vi "Teleop.vi"(10 "Match Info":T1={"Autonomous Elapsed Seconds"=0.0, "TeleOp Elapsed Seconds"=0.0, "Disabled Elapsed Seconds"=0.0, "Visited Autonomous"=FALSE, "Visited TeleOp"=FALSE, "Visited Disabled"=FALSE, "Autonomous Settings"={"Autonomous Style"=enum."Independent", "VI Refnum"=refnum}}, 11 "Call Context":T2) -> ()   [LabVIEW 2012]
doc: "This VI is called for each TeleOp packet received from the DS where the robot is not disabled. It is often used to read from the joysticks and update I/O or to update setpoints for timed control loops. It should complete and return within 20 milliseconds or it may miss DS packets."
uses:
  <vilib>/Rock Robotics/WPI/DriverStation/WPI_DriverStationDerivedRobotMode.ctl
  <vilib>/Rock Robotics/WPI/DriverStation/WPI_DriverStationMatch Info.ctl
  <vilib>/Rock Robotics/WPI/Relay/WPI_RelayValue.ctl
  Robot Global Data.vi
  <vilib>/Rock Robotics/WPI/Joystick/WPI_JoystickGetSetRefNum.vi
panel:
  in  "Numeric":dbl=0.87
  in  "Ext Const":dbl=0.5
  in  "Dep Const":dbl=1.0
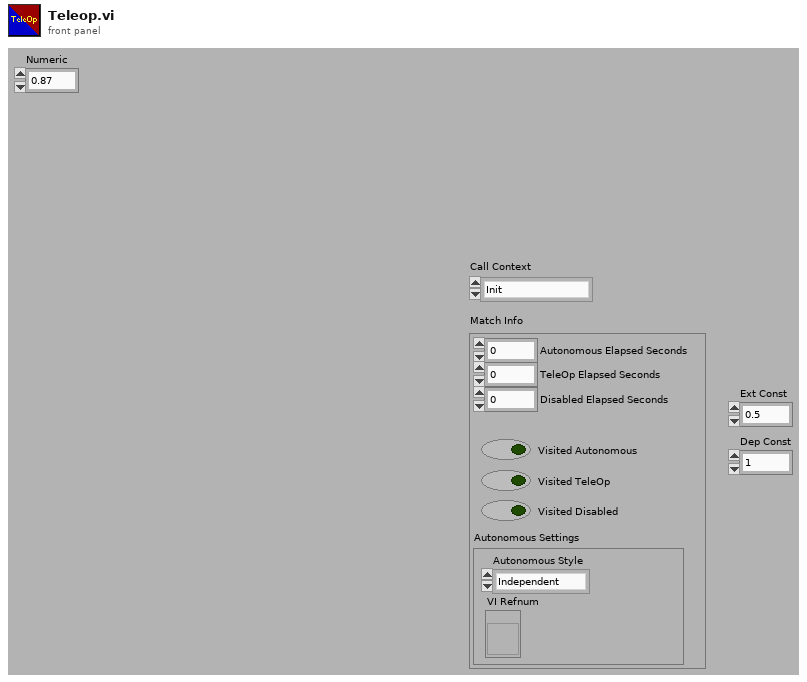
[diagram p1: front panel]
types:
  T1 = typedef "WPI_DriverStationMatch Info.ctl" = cluster{"Autonomous Elapsed Seconds":dbl, "TeleOp Elapsed Seconds":dbl, "Disabled Elapsed Seconds":dbl, "Visited Autonomous":bool, "Visited TeleOp":bool, "Visited Disabled":bool, "Autonomous Settings":cluster{"Autonomous Style":enum16{"Iterative", "Independent"}, "VI Refnum":refnum<vi>}}
  T2 = typedef "WPI_DriverStationDerivedRobotMode.ctl" = enum16{"Init", "Execute", "Stop"}
  T3 = typedef "WPI_RelayValue.ctl" = enum16{"Off", "On", "Forward", "Reverse"}
  T4 = cluster{"Driver Station Digital Input (1-8)[0]":bool, "Driver Station Digital Input (1-8)[1]":bool, "Driver Station Digital Input (1-8)[2]":bool, "Driver Station Digital Input (1-8)[3]":bool, "Driver Station Digital Input (1-8)[4]":bool, "Driver Station Digital Input (1-8)[5]":bool, "Driver Station Digital Input (1-8)[6]":bool, "Driver Station Digital Input (1-8)[7]":bool, "Driver Station Digital Input (1-8)[8]":bool}
  T5 = typedef "WPI_DigitalInputDevRef.ctl" = cluster{"DevStatus":errorcluster, "DIO Channel":T6, "Digital Module":T7}
  T6 = typedef "FPGA_DIOChannel.ctl" = enum8{"DIO 1", "DIO 2", "DIO 3", "DIO 4", "DIO 5", "DIO 6", "DIO 7", "DIO 8", "DIO 9", "DIO 10", "DIO 11", "DIO 12", "DIO 13", "DIO 14", "Invalid"}
  T7 = typedef "FPGA_TypedefDigitalModule.ctl" = enum16{"Digital Module 1", "Digital Module 2"}
  T8 = cluster{"Right Servo High":dbl, "Right Servo Mid":dbl, "Right Servo Low":dbl, "Left Servo High":dbl, "Left Servo Mid":dbl, "Left Servo Low":dbl}
  T9 = typedef "WPI_JoystickDevRef.ctl" = cluster{"Device":T10}
  T10 = typedef "WPI_JoystickDeviceEnum.ctl" = enum16{"USB 1", "USB 2", "USB 3", "USB 4", "Kinect 1", "Kinect 2"}
  T11 = cluster{"axis 1 (x)":dbl, "axis 2 (y)":dbl, "axis 3 (throttle)":dbl, "axis 4":dbl, "axis 5":dbl, "axis 6":dbl}
  T12 = typedef "WPI_ServoDeviceRef.ctl" = cluster{"DeviceStatus":errorcluster, "Digital Module":T7, "PWM Channel":T13, "DeadBand":T14}
  T13 = typedef "FPGA_DIOPWMChannel.ctl" = enum8{"PWM 1", "PWM 2", "PWM 3", "PWM 4", "PWM 5", "PWM 6", "PWM 7", "PWM 8", "PWM 9", "PWM 10", "Invalid"}
  T14 = typedef "WPI_PWMDeadband.ctl" = cluster{"Name":string, "maxPositivePwm":i32, "minPositivePwm":i32, "centerPwm":i32, "maxNegativePwm":i32, "minNegativePwm":i32, "angularRange":u16}
  T15 = typedef "WPI_RelayDevRef.ctl" = cluster{"DevStatus":errorcluster, "Relay Channel":T16, "Digital Module":T7, "Relay Direction":T17}
  T16 = typedef "FPGA_DIORelayChannel.ctl" = enum8{"Relay 1", "Relay 2", "Relay 3", "Relay 4", "Relay 5", "Relay 6", "Relay 7", "Relay 8", "Invalid"}
  T17 = typedef "WPI_RelayDirection.ctl" = enum16{"Both directions", "Forward only", "Reverse only"}
  T18 = typedef "WPI_MotorControlDeviceRef.ctl" = cluster{"DeviceStatus":errorcluster, "Type":enum16{"PWM", "CAN"}, "PWM":cluster{"Digital Module":T7, "PWM Channel":T13, "DeadBand":T14}, "CAN":cluster{"Device Number":u8, "Control Mode":T19, "Semaphore":T20, "Max Vout":dbl}, "Invert":bool, "TransformRef":T21, "InvTransformRef":T21}
  T19 = typedef "WPI_CANJaguar_ControlMode.ctl" = enum8{"Percent VBus", "Current", "Speed", "Position", "Voltage"}
  T20 = typedef "Semaphore RefNum" = refnum<k1>
  T21 = typedef "WPI_PWMTransform_ConPane.ctl" = refnum<vi>
  T22 = typedef "WPI_JoystickButtonState.ctl" = cluster{"Button 1":bool, "Button 2":bool, "Button 3":bool, "Button 4":bool, "Button 5":bool, "Button 6":bool, "Button 7":bool, "Button 8":bool, "Button 9":bool, "Button 10":bool, "Button 11":bool, "Button 12":bool}
  T23 = cluster{"FlipperLeftUp":dbl, "FlipperLeftDown":dbl, "FlipperRightUp":dbl, "FlipperRightDown":dbl, "KickerLeftBack":dbl, "KickerLeftForward":dbl, "KickerRightBack":dbl, "KickerRightForward":dbl}
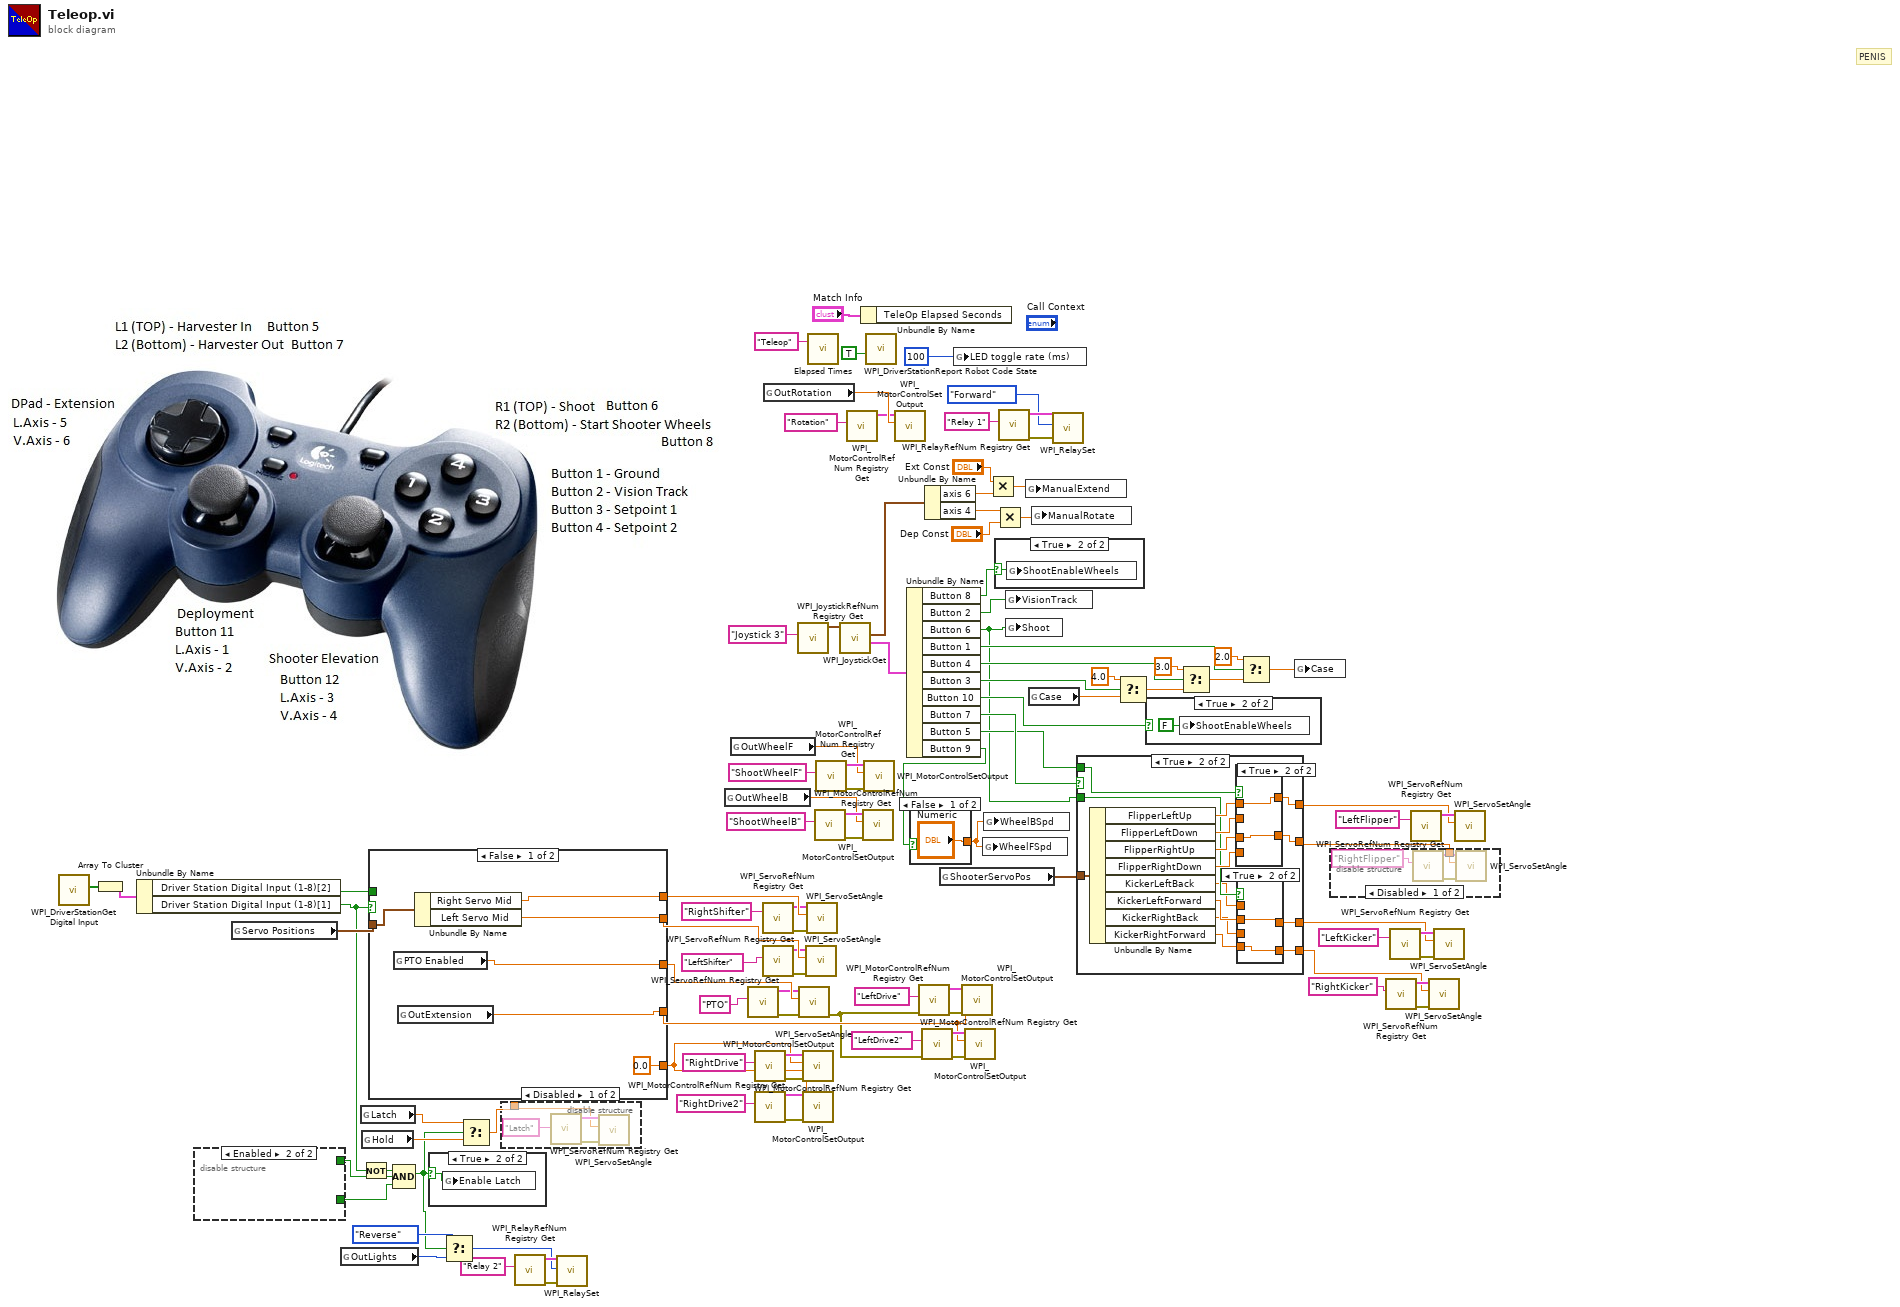
[diagram p0: block diagram]
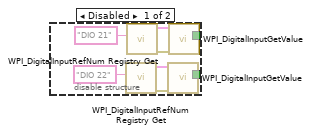
[diagram p2: hidden frame]
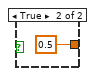
[diagram p4: hidden frame]
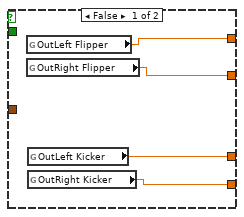
[diagram p6: hidden frame]
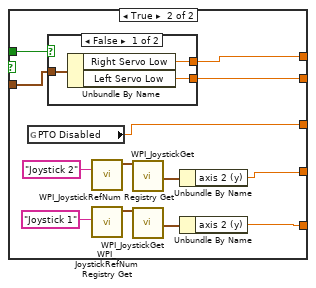
[diagram p10: hidden frame]
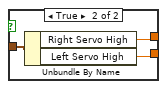
[diagram p11: hidden frame]
diagram:
  # "PENIS"
  n1 = call <vilib>:"WPI_DriverStationGet Digital Input.vi"() -> ("Driver Station Digital Input (1-8)"=w73:bool[])  [unwired: 11 in]
  n2 = Array To Cluster(array=w73) -> (cluster=w72:T4)
  n3 = Unbundle By Name(w72) -> ("Driver Station Digital Input (1-8)[2]"=w71:bool, "Driver Station Digital Input (1-8)[1]"=w35:bool)
  n4 = disable-structure shown="Enabled" {
    disable-tunnel: [w107 _] -> w3
    disable-tunnel: [w106 _] -> w2
    frame Disabled {
      n5 = call <vilib>:"WPI_DigitalInputRefNum Registry Get.vi"("refnum name"="DIO 22") -> ("error out"=w108:errorcluster, "DigitalInputDevRef"=w109:T5)  [unwired: 9 in]
      n6 = call <vilib>:"WPI_DigitalInputRefNum Registry Get.vi"("refnum name"="DIO 21") -> ("error out"=w113:errorcluster, "DigitalInputDevRef"=w112:T5)  [unwired: 9 in]
      n7 = call <vilib>:"WPI_DigitalInputGetValue.vi"("error in (no error)"=w108, "DigitalInputDevRef"=w109) -> ("Value"=w106:bool)  [unwired: 7 in, 2 out]
      n8 = call <vilib>:"WPI_DigitalInputGetValue.vi"("error in (no error)"=w113, "DigitalInputDevRef"=w112) -> ("Value"=w107:bool)  [unwired: 7 in, 2 out]
    }
    frame Enabled {
    }
  }
  n9 = global read "Robot Global Data.vi" "Servo Positions"() -> (w70:T8)
  n10 = global read "Robot Global Data.vi" "OutLights"() -> (w38:T3)
  n11 = global read "Robot Global Data.vi" "Latch"() -> (w8:dbl)
  n12 = Not(x=w35) -> (.not. x?=w4:bool)
  n13 = global read "Robot Global Data.vi" "Hold"() -> (w7:dbl)
  n14 = case shown="False" w35 {
    tunnel: w71 -> [_ w132]
    tunnel: w70 -> [w119 w131]
    tunnel: [w118 w130] -> w69
    tunnel: [w117 w129] -> w68
    tunnel: [w116 w128] -> w61
    tunnel: [w114 w121] -> w60
    tunnel: [0.0 w120] -> w59
    frame False {
      n15 = global read "Robot Global Data.vi" "PTO Enabled"() -> (w116:dbl)
      n16 = global read "Robot Global Data.vi" "OutExtension"() -> (w114:dbl)
      n17 = Unbundle By Name(w119) -> ("Right Servo Mid"=w118:dbl, "Left Servo Mid"=w117:dbl)
    }
    frame True {
      n18 = global read "Robot Global Data.vi" "PTO Disabled"() -> (w128:dbl)
      n19 = case shown="False" w132 {
        tunnel: w131 -> [w135 w138]
        tunnel: [w134 w137] -> w130
        tunnel: [w133 w136] -> w129
        frame False {
          n20 = Unbundle By Name(w135) -> ("Right Servo Low"=w134:dbl, "Left Servo Low"=w133:dbl)
        }
        frame True {
          n21 = Unbundle By Name(w138) -> ("Right Servo High"=w137:dbl, "Left Servo High"=w136:dbl)
        }
      }
      n22 = call <vilib>:"WPI_JoystickRefNum Registry Get.vi"("refnum name"="Joystick 2") -> ("JoystickDevRef"=w122:T9)  [unwired: 1 in, 9 out]
      n23 = call <vilib>:"WPI_JoystickRefNum Registry Get.vi"("refnum name"="Joystick 1") -> ("JoystickDevRef"=w126:T9)  [unwired: 1 in, 9 out]
      n24 = call <vilib>:"WPI_JoystickGet.vi"("JoystickDevRef"=w122) -> ("Axes"=w124:T11)  [unwired: 1 in, 5 out]
      n25 = call <vilib>:"WPI_JoystickGet.vi"("JoystickDevRef"=w126) -> ("Axes"=w127:T11)  [unwired: 1 in, 5 out]
      n26 = Unbundle By Name(w124) -> ("axis 2 (y)"=w121:dbl)
      n27 = Unbundle By Name(w127) -> ("axis 2 (y)"=w120:dbl)
    }
  }
  n28 = Compound Arithmetic op=AND(w4, w3, w2) -> (w1:bool)
  n29 = case shown="True" w1 {
    selector: w1 -> [_ w139]
    frame False {
    }
    frame True {
      n30 = global write "Robot Global Data.vi" "Enable Latch"(w139) -> ()
    }
  }
  n31 = Select(t=WPI_RelayValue."Reverse" ("RelayValue"), s=w1, f=w38) -> (s? t:f=w36:T3)
  n32 = Select(t=w8, s=w1, f=w7) -> (s? t:f=w34:dbl)
  n33 = disable-structure shown="Disabled" {
    disable-tunnel: w34 -> [w140 _]
    frame Disabled {
      n34 = call <vilib>:"WPI_ServoRefNum Registry Get.vi"("refnum name"="Latch") -> ("error out"=w143:errorcluster, "ServoDeviceRef"=w141:T12)  [unwired: 9 in]
      n35 = call <vilib>:"WPI_ServoSetAngle.vi"("error in (no error)"=w143, "Angle"=w140, "ServoDeviceRef"=w141) -> ()  [unwired: 7 in, 2 out]
    }
    frame Enabled {
    }
  }
  n36 = call <vilib>:"WPI_RelayRefNum Registry Get.vi"("refnum name"="Relay 2") -> ("error out"=w44:errorcluster, "RelayDevRef"=w42:T15)  [unwired: 9 in]
  n37 = call <vilib>:"WPI_RelaySet.vi"("error in (no error)"=w44, "RelayValue"=w36, "RelayDevRef"=w42) -> ()  [unwired: 7 in, 2 out]
  n38 = global read "Robot Global Data.vi" "OutWheelB"() -> (w26:dbl)
  n39 = global read "Robot Global Data.vi" "OutWheelF"() -> (w27:dbl)
  n40 = call <vilib>:"WPI_ServoRefNum Registry Get.vi"("refnum name"="PTO") -> ("error out"=w54:errorcluster, "ServoDeviceRef"=w55:T12)  [unwired: 9 in]
  n41 = call <vilib>:"WPI_MotorControlRefNum Registry Get.vi"("refnum name"="RightDrive") -> ("error out"=w83:errorcluster, "MotorControlDevRef"=w85:T18)  [unwired: 9 in]
  n42 = call <vilib>:"WPI_MotorControlRefNum Registry Get.vi"("refnum name"="RightDrive2") -> ("error out"=w76:errorcluster, "MotorControlDevRef"=w74:T18)  [unwired: 9 in]
  n43 = call <vilib>:"WPI_ServoRefNum Registry Get.vi"("refnum name"="RightShifter") -> ("error out"=w64:errorcluster, "ServoDeviceRef"=w65:T12)  [unwired: 9 in]
  n44 = call <vilib>:"WPI_ServoRefNum Registry Get.vi"("refnum name"="LeftShifter") -> ("error out"=w66:errorcluster, "ServoDeviceRef"=w67:T12)  [unwired: 9 in]
  n45 = global read "Robot Global Data.vi" "OutRotation"() -> (w58:dbl)
  n46 = call <vilib>:"WPI_JoystickRefNum Registry Get.vi"("refnum name"="Joystick 3") -> ("JoystickDevRef"=w102:T9)  [unwired: 9 in, 1 out]
  n47 = call <vilib>:"WPI_ServoSetAngle.vi"("error in (no error)"=w54, "Angle"=w61, "ServoDeviceRef"=w55) -> ("error out"=w50:errorcluster)  [unwired: 7 in, 1 out]
  n48 = call <vilib>:"WPI_MotorControlSetOutput.vi"("error in (no error)"=w83, "Output"=w59, "MotorControlDevRef"=w85) -> ()  [unwired: 6 in, 3 out]
  n49 = call <vilib>:"WPI_MotorControlSetOutput.vi"("error in (no error)"=w76, "Output"=w59, "MotorControlDevRef"=w74) -> ()  [unwired: 6 in, 3 out]
  n50 = call <vilib>:"WPI_ServoSetAngle.vi"("error in (no error)"=w66, "Angle"=w68, "ServoDeviceRef"=w67) -> ()  [unwired: 7 in, 2 out]
  n51 = call <vilib>:"WPI_ServoSetAngle.vi"("error in (no error)"=w64, "Angle"=w69, "ServoDeviceRef"=w65) -> ()  [unwired: 7 in, 2 out]
  n52 = call "Elapsed Times.vi"("Call Name"="Teleop") -> ()  [unwired: 2 in, 1 out]
  n53 = call <vilib>:"WPI_MotorControlRefNum Registry Get.vi"("refnum name"="ShootWheelB") -> ("error out"=w29:errorcluster, "MotorControlDevRef"=w30:T18)  [unwired: 9 in]
  n54 = call <vilib>:"WPI_MotorControlRefNum Registry Get.vi"("refnum name"="ShootWheelF") -> ("error out"=w31:errorcluster, "MotorControlDevRef"=w28:T18)  [unwired: 9 in]
  n55 = call <vilib>:"WPI_JoystickGet.vi"("JoystickDevRef"=w102) -> ("Buttons"=w100:T22, "Axes"=w99:T11)  [unwired: 4 in, 1 out]
  n56 = call <vilib>:"WPI_MotorControlRefNum Registry Get.vi"("refnum name"="Rotation") -> ("MotorControlDevRef"=w56:T18)  [unwired: 9 in, 1 out]
  n57 = Unbundle By Name("Match Info") -> ()  [unwired: 1 out]
  n58 = call <vilib>:"WPI_MotorControlSetOutput.vi"("error in (no error)"=w29, "Output"=w26, "MotorControlDevRef"=w30) -> ()  [unwired: 6 in, 3 out]
  n59 = call <vilib>:"WPI_MotorControlSetOutput.vi"("error in (no error)"=w31, "Output"=w27, "MotorControlDevRef"=w28) -> ()  [unwired: 6 in, 3 out]
  n60 = call <vilib>:"WPI_DriverStationReport Robot Code State.vi"("TeleOp"=TRUE ("Autonomous")) -> ()  [unwired: 10 in, 1 out]
  n61 = call <vilib>:"WPI_MotorControlSetOutput.vi"("Output"=w58, "MotorControlDevRef"=w56) -> ()  [unwired: 7 in, 3 out]
  n62 = Unbundle By Name(w100) -> ("Button 8"=w87:bool, "Button 2"=w98:bool, "Button 6"=w10:bool, "Button 1"=w97:bool, "Button 4"=w95:bool, "Button 3"=w94:bool, "Button 10"=w25:bool, "Button 7"=w24:bool, "Button 5"=w23:bool, "Button 9"=w5:bool)
  n63 = case shown="False" w5 {
    tunnel: ["Numeric" 0.5] -> w6
    frame False {
    }
    frame True {
    }
  }
  n64 = call <vilib>:"WPI_MotorControlRefNum Registry Get.vi"("error in (no error)"=w50, "refnum name"="LeftDrive") -> ("error out"=w78:errorcluster, "MotorControlDevRef"=w81:T18)  [unwired: 8 in]
  n65 = call <vilib>:"WPI_MotorControlRefNum Registry Get.vi"("error in (no error)"=w50, "refnum name"="LeftDrive2") -> ("error out"=w77:errorcluster, "MotorControlDevRef"=w79:T18)  [unwired: 8 in]
  n66 = Unbundle By Name(w99) -> ("axis 6"=w41:dbl, "axis 4"=w51:dbl)
  n67 = global read "Robot Global Data.vi" "ShooterServoPos"() -> (w11:T23)
  n68 = global write "Robot Global Data.vi" "LED toggle rate (ms)"(u32 100 ("LED ms toggle rate")) -> ()
  n69 = call <vilib>:"WPI_MotorControlSetOutput.vi"("error in (no error)"=w78, "Output"=w60, "MotorControlDevRef"=w81) -> ()  [unwired: 6 in, 3 out]
  n70 = call <vilib>:"WPI_MotorControlSetOutput.vi"("error in (no error)"=w77, "Output"=w60, "MotorControlDevRef"=w79) -> ()  [unwired: 6 in, 3 out]
  n71 = global write "Robot Global Data.vi" "WheelFSpd"(w6) -> ()
  n72 = global write "Robot Global Data.vi" "WheelBSpd"(w6) -> ()
  n73 = Multiply(x="Ext Const", y=w41) -> (x*y=w39:dbl)
  n74 = Multiply(x=w51, y="Dep Const") -> (x*y=w49:dbl)
  n75 = case shown="True" w87 {
    selector: w87 -> [_ w146]
    frame False {
    }
    frame True {
      n76 = global write "Robot Global Data.vi" "ShootEnableWheels"(w146) -> ()
    }
  }
  n77 = call <vilib>:"WPI_RelayRefNum Registry Get.vi"("refnum name"="Relay 1") -> ("error out"=w46:errorcluster, "RelayDevRef"=w48:T15)  [unwired: 9 in]
  n78 = global write "Robot Global Data.vi" "VisionTrack"(w98) -> ()
  n79 = global write "Robot Global Data.vi" "Shoot"(w10) -> ()
  n80 = global write "Robot Global Data.vi" "ManualExtend"(w39) -> ()
  n81 = global read "Robot Global Data.vi" "Case"() -> (w89:dbl)
  n82 = global write "Robot Global Data.vi" "ManualRotate"(w49) -> ()
  n83 = call <vilib>:"WPI_RelaySet.vi"("error in (no error)"=w46, "RelayValue"=WPI_RelayValue."Forward", "RelayDevRef"=w48) -> ()  [unwired: 7 in, 2 out]
  n84 = case shown="True" w24 {
    tunnel: w23 -> [_ w151]
    tunnel: [w150 w164] -> w14
    tunnel: [w149 w162] -> w13
    tunnel: [w148 w153] -> w12
    tunnel: [w147 w152] -> w9
    tunnel: w11 -> [_ w165]
    tunnel: w10 -> [_ w158]
    frame False {
      n85 = global read "Robot Global Data.vi" "OutLeft Flipper"() -> (w150:dbl)
      n86 = global read "Robot Global Data.vi" "OutRight Flipper"() -> (w149:dbl)
      n87 = global read "Robot Global Data.vi" "OutLeft Kicker"() -> (w148:dbl)
      n88 = global read "Robot Global Data.vi" "OutRight Kicker"() -> (w147:dbl)
    }
    frame True {
      n89 = Unbundle By Name(w165) -> ("FlipperLeftUp"=w163:dbl, "FlipperLeftDown"=w160:dbl, "FlipperRightUp"=w161:dbl, "FlipperRightDown"=w159:dbl, "KickerLeftBack"=w157:dbl, "KickerLeftForward"=w156:dbl, "KickerRightBack"=w155:dbl, "KickerRightForward"=w154:dbl)
      n90 = case shown="True" w151 {
        tunnel: [w171 w173] -> w164
        tunnel: w163 -> [_ w173]
        tunnel: [w170 w172] -> w162
        tunnel: w161 -> [_ w172]
        tunnel: w160 -> [w171 _]
        tunnel: w159 -> [w170 _]
        frame False {
        }
        frame True {
        }
      }
      n91 = case shown="True" w158 {
        tunnel: w157 -> [w167 _]
        tunnel: w156 -> [_ w168]
        tunnel: w155 -> [w166 _]
        tunnel: w154 -> [_ w169]
        tunnel: [w167 w168] -> w153
        tunnel: [w166 w169] -> w152
        frame False {
        }
        frame True {
        }
      }
    }
  }
  n92 = Select(t=4.0, s=w94, f=w89) -> (s? t:f=w93:dbl)
  n93 = case shown="True" w25 {
    frame False {
    }
    frame True {
      n94 = global write "Robot Global Data.vi" "ShootEnableWheels"(FALSE ("ShootStartWheels")) -> ()
    }
  }
  n95 = Select(t=3.0, s=w95, f=w93) -> (s? t:f=w91:dbl)
  n96 = Select(t=2.0, s=w97, f=w91) -> (s? t:f=w88:dbl)
  n97 = global write "Robot Global Data.vi" "Case"(w88) -> ()
  n98 = disable-structure shown="Disabled" {
    disable-tunnel: w13 -> [w175 _]
    frame Disabled {
      n99 = call <vilib>:"WPI_ServoRefNum Registry Get.vi"("refnum name"="RightFlipper") -> ("error out"=w178:errorcluster, "ServoDeviceRef"=w176:T12)  [unwired: 9 in]
      n100 = call <vilib>:"WPI_ServoSetAngle.vi"("error in (no error)"=w178, "Angle"=w175, "ServoDeviceRef"=w176) -> ()  [unwired: 7 in, 2 out]
    }
    frame Enabled {
    }
  }
  n101 = call <vilib>:"WPI_ServoRefNum Registry Get.vi"("refnum name"="RightKicker") -> ("error out"=w21:errorcluster, "ServoDeviceRef"=w19:T12)  [unwired: 9 in]
  n102 = call <vilib>:"WPI_ServoRefNum Registry Get.vi"("refnum name"="LeftKicker") -> ("error out"=w15:errorcluster, "ServoDeviceRef"=w16:T12)  [unwired: 9 in]
  n103 = call <vilib>:"WPI_ServoRefNum Registry Get.vi"("refnum name"="LeftFlipper") -> ("ServoDeviceRef"=w17:T12)  [unwired: 9 in, 1 out]
  n104 = call <vilib>:"WPI_ServoSetAngle.vi"("error in (no error)"=w21, "Angle"=w9, "ServoDeviceRef"=w19) -> ()  [unwired: 7 in, 2 out]
  n105 = call <vilib>:"WPI_ServoSetAngle.vi"("error in (no error)"=w15, "Angle"=w12, "ServoDeviceRef"=w16) -> ()  [unwired: 7 in, 2 out]
  n106 = call <vilib>:"WPI_ServoSetAngle.vi"("Angle"=w14, "ServoDeviceRef"=w17) -> ()  [unwired: 8 in, 2 out]
